vi "Actor Core.vi"(8 "error in":errorcluster, 11 "SAS_AFTester_Template in":refnum<class "Business Logic Tester.lvclass">) -> (0 "error out":errorcluster, 3 "Actor out":refnum<class "Actor.lvclass">)   [LabVIEW 2020, in "Business Logic Tester.lvlib" / "Business Logic Tester.lvclass"]
doc: "(<B>Filename</B>: Actor Framework.lvlib:Actor.lvclass:Actor Core.vi)\n\nReceives messages to the actor, reacts to them, and initiates any error handling that may shut the actor down.\n\nDescendant classes may override this VI to append parallel tasks for the actor to complete while it handles messages. Overrides use the Call Parent Method node."
uses:
  Business Logic Tester.lvclass
  C:/Program Files (x86)/National Instruments/LabVIEW 2020/vi.lib/ActorFramework/Actor/Actor.lvclass
  <vilib>/ActorFramework/Actor/Actor.lvclass
  <vilib>/Utility/miscctls.llb/LVPointTypeDef.ctl
  <vilib>/ActorFramework/Actor/Actor.lvclass/Actor.ctl
  <vilib>/ActorFramework/Message Enqueuer/Message Enqueuer.lvclass/Message Enqueuer.ctl
  Business Logic Tester.lvclass/Business Logic Tester.ctl
  Business Logic Tester Messages/To AUT Stop Msg/To AUT Stop Msg.lvclass/To AUT Stop Msg.ctl
  Business Logic Tester Messages/To AUT Error Msg/To AUT Error Msg.lvclass/To AUT Error Msg.ctl
  <vilib>/ActorFramework/Report Error Msg/Report Error Msg.lvclass/Report Error Msg.ctl
  <vilib>/ActorFramework/Message Enqueuer/Init from Existing Queue.vi
  <vilib>/ActorFramework/Message Enqueuer/Enqueue.vi
  <vilib>/ActorFramework/Stop Msg/Stop Msg.lvclass
  C:/Program Files (x86)/National Instruments/LabVIEW 2020/vi.lib/ActorFramework/Message/Message.lvclass
  Business Logic Tester Messages/To AUT Stop Msg/To AUT Stop Msg.lvclass
  Business Logic Tester Messages/To AUT Error Msg/To AUT Error Msg.lvclass
  Business Logic Tester Messages/Launch New AUT Instance Msg/Launch New AUT Instance Msg.lvclass
  <vilib>/ActorFramework/Report Error Msg/Report Error Msg.lvclass
  <vilib>/ActorFramework/Message Priority Queue/Priority Enqueue.vi
  <vilib>/ActorFramework/Message Enqueuer/Message Enqueuer.lvclass
panel:
  in  "Send Error Button":bool
  out "Total Active  Instances":i32=1 min=1 step=1
  in  "# to Launch":i32=1 min=1 step=1
  out "AFTester_Label":string
  in  "Save Log Button":bool
  in  "Clear Log Button":bool
  in  "Stop Instance":bool
  out "Active Instances":string[](array[string])
  in  "Instance to Send Message To":u16(ring)
  in  "Launch New Instance Button":bool
  out "Log":string
  in  "Exit Tester Button":bool
  # "Unplaced Controls"
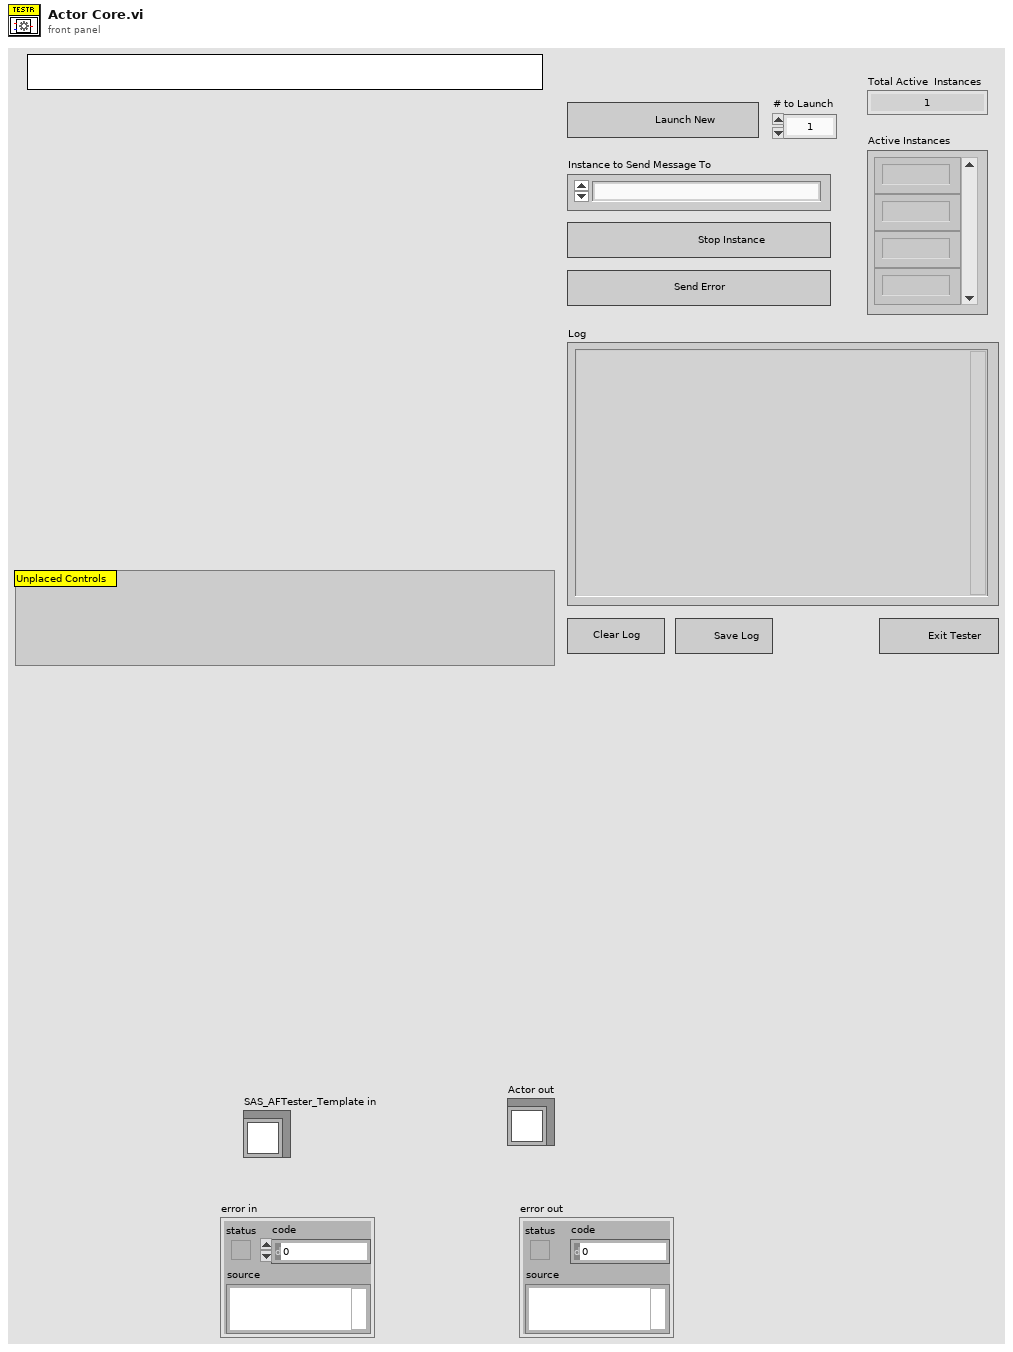
[diagram p1: front panel]
types:
  T1 = typedef "LVPointTypeDef.ctl" = cluster{"Horizontal":i16, "Vertical":i16}
  T2 = enum32{"Invalid", "Standard", "Closed", "Hidden", "Minimized", "Maximized"}
  T3 = typedef "Business Logic Tester.lvlib/Business Logic Tester.lvclass/Events for GUI.ctl" = cluster{"Stop Event":refnum<user-event>, "Log Event":refnum<user-event>, "Active Modules Event":refnum<user-event>}
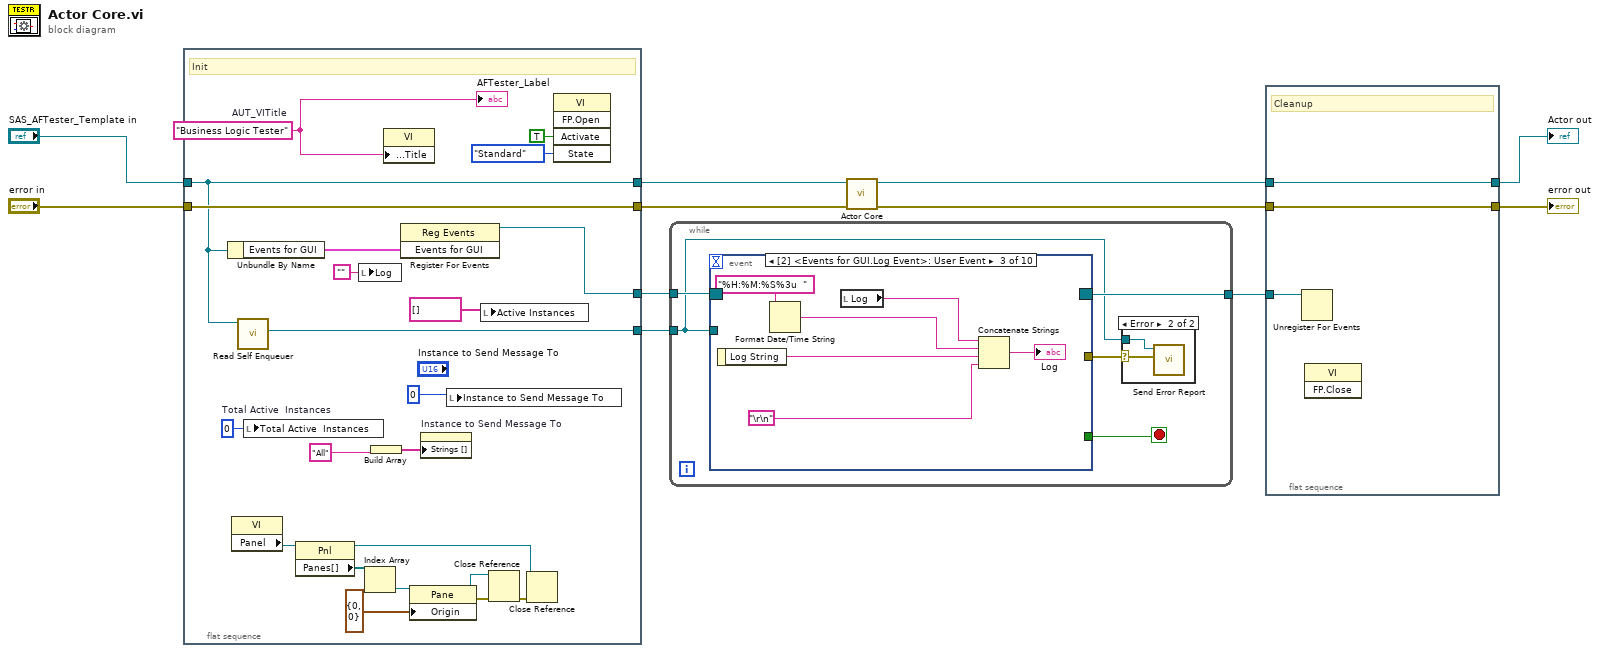
[diagram p0: block diagram]
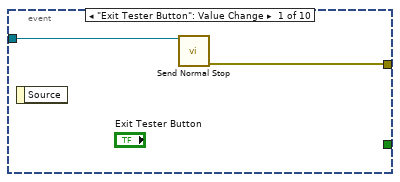
[diagram p3: hidden frame]
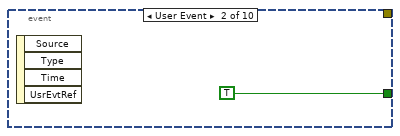
[diagram p4: hidden frame]
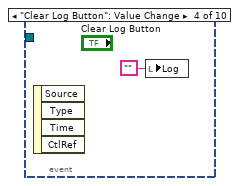
[diagram p5: hidden frame]
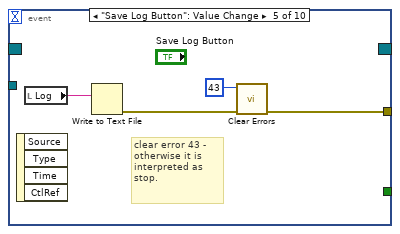
[diagram p6: hidden frame]
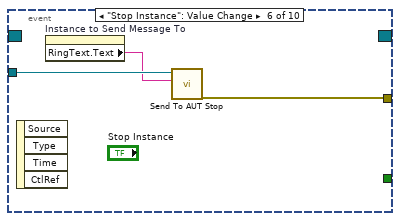
[diagram p7: hidden frame]
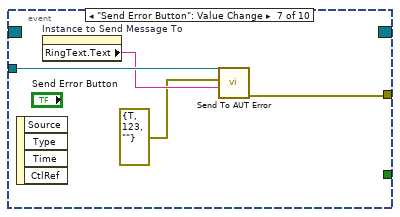
[diagram p8: hidden frame]
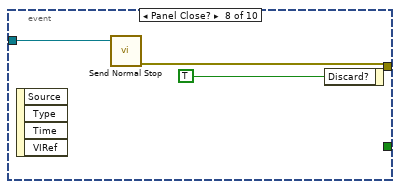
[diagram p9: hidden frame]
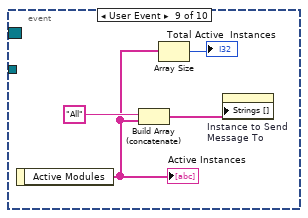
[diagram p10: hidden frame]
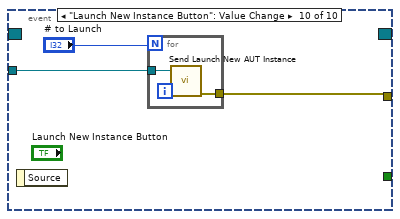
[diagram p11: hidden frame]
diagram:
  n1 = flat-sequence {
    tunnel: [w31] -> w10
    tunnel: "SAS_AFTester_Template in" -> [w31]
    tunnel: "error in" -> [w33]
    tunnel: [w33] -> w9
    tunnel: [w32] -> w3
    tunnel: [w30] -> w2
    frame #0 {
      w21 = 0  # Total Active  Instances
      w20 = "Business Logic Tester"  # AUT_VITitle
      # "Init"
      n2 = Unbundle By Name(w31) -> ("Events for GUI"=w27:T3)
      n3 = property class="VI"() -> ("Panel"=w19:refnum<vi>)  [unwired: 2 in, 2 out]
      n4 = call <vilib>:"Read Self Enqueuer.vi"("Actor"=w31) -> ("Self Enqueuer"=w30:refnum<class "Message Enqueuer.lvclass">)  [unwired: 10 in]
      n5 = local write "Total Active  Instances"(w21) -> ()
      n6 = property class="Pnl"(reference=w19) -> (reference out=w12:refnum<vi>, "Panes[]"=w18:refnum<vi>[])  [unwired: 1 in, 1 out]
      n7 = local write "Log"("" ("Log")) -> ()
      n8 = Index Array(array=w18) -> (element=w17:refnum<vi>)  [unwired: 1 in]
      n9 = Build Array("All" ("string")) -> (w25:string[])
      n10 = property class="VI"("Front Panel.Title"=w20) -> ()  [unwired: 2 in, 2 out]
      n11 = register-events(w27) -> (reference out=w32:refnum<event-registration>)  [unwired: 2 in, 1 out]
      n12 = property class="Pane"(reference=w17, "Origin"=T1 {"Horizontal"=0, "Vertical"=0}) -> (reference out=w14:refnum<vi>, error out=w15:errorcluster)  [unwired: 1 in]
      n13 = property on="Instance to Send Message To" class="Ring (strict)"("Strings []"=w25) -> ()  [unwired: 2 in, 2 out]
      n14 = local write "Instance to Send Message To"(0) -> ()
      n15 = local write "Active Instances"(string[] [] ("Active Modules")) -> ()
      n16 = Close Reference(reference=w14, error in (no error)=w15) -> (error out=w13:errorcluster)
      n17 = Close Reference(reference=w12, error in (no error)=w13) -> ()  [unwired: 1 out]
      n18 = invoke class="VI" method="FP.Open"("Activate"=TRUE ("Activate?"), "State"=T2."Standard") -> ()  [unwired: 3 in, 5 out]
      "AFTester_Label" <- w20
    }
  }
  n19 = while {
    tunnel: w3 -> [w38]
    tunnel: w2 -> [w34]
    tunnel: [w36] -> w1
    stop <- w37 stop-if-true
    n20 = event shown="[2] <Events for GUI.Log Event>: User Event" {
      selector: w38 -> [_ _ _ _ _ _ _ _ _ _]
      dyn-events: [_ _ _ _ _ _ _ _ _ _] -> w36
      timeout: _ -> [_ _ _ _ _ _ _ _ _ _]
      tunnel: w34 -> [w42 _ _ _ _ w57 w61 w63 _ w71]
      tunnel: [_ TRUE _ _ _ _ _ _ _ _] -> w37
      tunnel: [w41 _ _ _ w51 w55 w60 w62 _ w70] -> w35
      event "Exit Tester Button": Value Change {
        n21 = event-data() -> ()  [unwired: 1 in, 1 out]
        n22 = call <vilib>:"Send Normal Stop.vi"("Message Enqueuer"=w42) -> ("error out"=w41:errorcluster)  [unwired: 10 in]
      }
      event User Event {
        n23 = event-data() -> ()  [unwired: 1 in, 4 out]
      }
      event User Event {
        n24 = event-data() -> ("Log String"=w49:string)  [unwired: 1 in]
        n25 = Format Date/Time String(time format string (%c)="%H:%M:%S%3u  ") -> (date/time string=w47:string)  [unwired: 2 in]
        n26 = local read "Log"() -> (w44:string)
        n27 = Concatenate Strings(w44, w47, w49, "\r\n" ("End of Line Constant")) -> (→"Log":string)
      }
      event "Clear Log Button": Value Change {
        n28 = event-data() -> ()  [unwired: 1 in, 4 out]
        n29 = local write "Log"("" ("Log")) -> ()
      }
      event "Save Log Button": Value Change {
        # "clear error 43 - otherwise it is interpreted as stop."
        n30 = event-data() -> ()  [unwired: 1 in, 4 out]
        n31 = local read "Log"() -> (w54:string)
        n32 = Write to Text File(text=w54) -> (error out=w52:errorcluster)  [unwired: 3 in, 2 out]
        n33 = call <vilib>:"Clear Errors.vi"("error in (no error)"=w52, "specific error code to clear (0: all)"=43 ("y")) -> ("error out"=w51:errorcluster)  [unwired: 4 in, 1 out]
      }
      event "Stop Instance": Value Change {
        n34 = event-data() -> ()  [unwired: 1 in, 4 out]
        n35 = property on="Instance to Send Message To" class="Ring (strict)"() -> ("RingText.Text"=w56:string)  [unwired: 2 in, 2 out]
        n36 = call "Send To AUT Stop.vi"("Enqueuer ID"=w56, "Message Enqueuer"=w57) -> ("error out"=w55:errorcluster)  [unwired: 8 in, 1 out]
      }
      event "Send Error Button": Value Change {
        n37 = event-data() -> ()  [unwired: 1 in, 4 out]
        n38 = property on="Instance to Send Message To" class="Ring (strict)"() -> ("RingText.Text"=w59:string)  [unwired: 2 in, 2 out]
        n39 = call "Send To AUT Error.vi"("Enqueuer ID"=w59, "Error to Send"=errorcluster {"status"=TRUE, "code"=123, "source"=""}, "Message Enqueuer"=w61) -> ("error out"=w60:errorcluster)  [unwired: 7 in, 1 out]
      }
      event Panel Close? {
        n40 = event-data() -> ()  [unwired: 1 in, 4 out]
        n41 = call <vilib>:"Send Normal Stop.vi"("Message Enqueuer"=w63) -> ("error out"=w62:errorcluster)  [unwired: 10 in]
        n42 = event-data("Discard?"=TRUE) -> ()  [unwired: 1 in, 1 out]
      }
      event User Event {
        n43 = event-data() -> ("Active Modules"=w65:string[])  [unwired: 1 in]
        "Active Instances" <- w65
        n44 = Build Array (concatenate)("All" ("string"), w65) -> (w67:string[])
        n45 = Array Size(array=w65) -> (size(s)=→"Total Active  Instances":i32)
        n46 = property on="Instance to Send Message To" class="Ring (strict)"("Strings []"=w67) -> ()  [unwired: 2 in, 2 out]
      }
      event "Launch New Instance Button": Value Change {
        n47 = event-data() -> ()  [unwired: 1 in, 1 out]
        n48 = for {
          N: "# to Launch" -> [_]
          tunnel: w71 -> [w73]
          tunnel: [w72] -> w70
          n49 = call "Send Launch New AUT Instance.vi"("Message Enqueuer"=w73) -> ("error out"=w72:errorcluster)  [unwired: 9 in, 1 out]
        }
      }
    }
    n50 = case shown="Error" w35 {
      selector: w35 -> [_ w39]
      tunnel: w34 -> [_ w40]
      frame No Error {
      }
      frame Error {
        n51 = call <vilib>:"Send Error Report.vi"("Error From Sender"=w39, "Message Enqueuer"=w40) -> ()  [unwired: 9 in, 1 out]
      }
    }
  }
  n52 = call-parent "Actor Core.vi"("error in"=w9, "Actor in"=w10) -> ("error out"=w5:errorcluster, "Actor out"=w7:refnum<class "Actor.lvclass">)  [unwired: 8 in]
  n53 = flat-sequence {
    tunnel: w7 -> [w76]
    tunnel: [w76] -> w6
    tunnel: w5 -> [w75]
    tunnel: [w75] -> w4
    tunnel: w1 -> [w74]
    frame #0 {
      # "Cleanup"
      n54 = Unregister For Events(event registration refnum=w74) -> ()  [unwired: 1 in, 1 out]
      n55 = invoke class="VI" method="FP.Close"() -> ()  [unwired: 3 in, 3 out]
    }
  }
  "error out" <- w4
  "Actor out" <- w6
